vi "Glimpse Image Display Controller.vi"() -> ()   [LabVIEW 2015]
doc: "This widget allows the user to separately adjust the properties of mulltiple, independently displayed image windows. The controller is a stand-alone VI that can run in a separate thread from the program that is producing the images, so that the image display settings can be adjusted whilst other things (e.g., data acquisition) are occurring simultaneously."
uses:
  Image to Display event.ctt
  <vilib>/vision/Image Controls.llb/IMAQ Image.ctl
  GLIMPSE Globals.vi
panel:
  in  "to window":i8=9 min=2 max=9 step=1
  in  "Snapshot":bool
  in  "Presets":T1(array[cluster])=[{"Mem"=FALSE, "Black"=-32500.0, "White"=-25000.0, "Recall"=FALSE}]
  in  "Keep this in corner?":bool=TRUE
  in  "Autosize M":bool
  in  "Autoposition M":bool
  in  "Autoscale M":bool
  in  "Zoom +":bool
  in  "Zoom -":bool
  out "In use":bool
  in  "Auto size":bool
  in  "Auto position":bool
  in  "Autoscale":bool
  out "Window Title":string
  in  "Control image window #":u8(slide)=1 max=1 step=1 scale=0.0..1.0
  out "error out":errorcluster
  out "Black/White Levels temp":cluster{ext, ext}(slide)={1.0, 65535.0} scale=-32767.0..327567.0
  in  "Black/White Levels":cluster{ext, ext}(slide)={1.0, 65535.0} scale=-32767.0..327567.0
  in  "Stop":bool
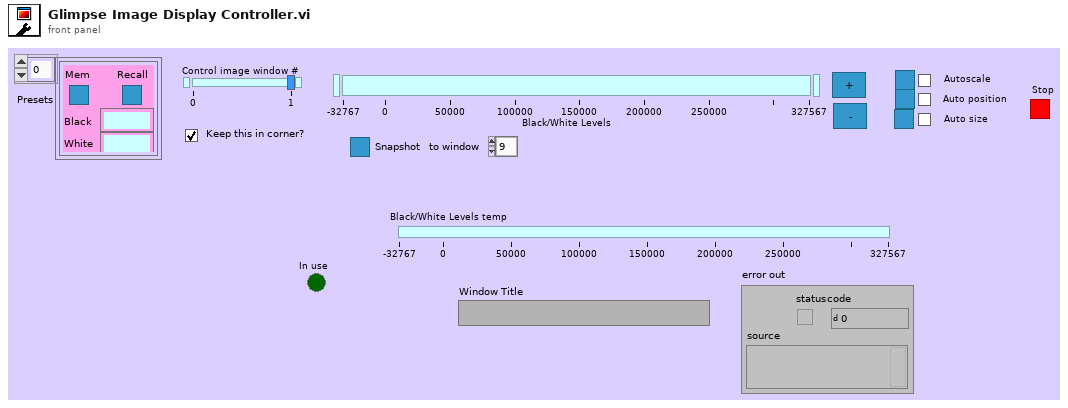
[diagram p1: front panel]
types:
  T1 = cluster{"Mem":bool, "Black":ext, "White":ext, "Recall":bool}[]
  T2 = typedef "Image Type" = u32
  T3 = typedef "IMAQ Image.ctl" = refnum<image>
  T4 = cluster{"Image Type":T2, "Image":T3, "Initialized?":bool, "Window Title":string, "Auto resize?":bool, "Auto position?":bool, "Autoscale?":bool, "Black/White Levels":cluster{ext, ext}, "Scale Min":ext, "Scale Max":ext}
  T5 = typedef "LVRectTypeDef.ctl" = cluster{"Left":i16, "Top":i16, "Right":i16, "Bottom":i16}
  T6 = typedef "Image to Display event.ctt" = cluster{"Image":T3, "Window Title":string, "Window Number":i32, "Image Type":T2, "Quit display controller?":bool}
  T7 = cluster{"Image Type":T2, "Image":T3, "Initialized?":bool, "Window Title":string, "Auto resize?":bool, "Auto position?":bool, "Autoscale?":bool, "Black/White Levels":cluster{ext, ext}, "Scale Min":ext, "Scale Max":ext}[]
  T8 = cluster{"Mem":bool, "Black":ext, "White":ext, "Recall":bool}
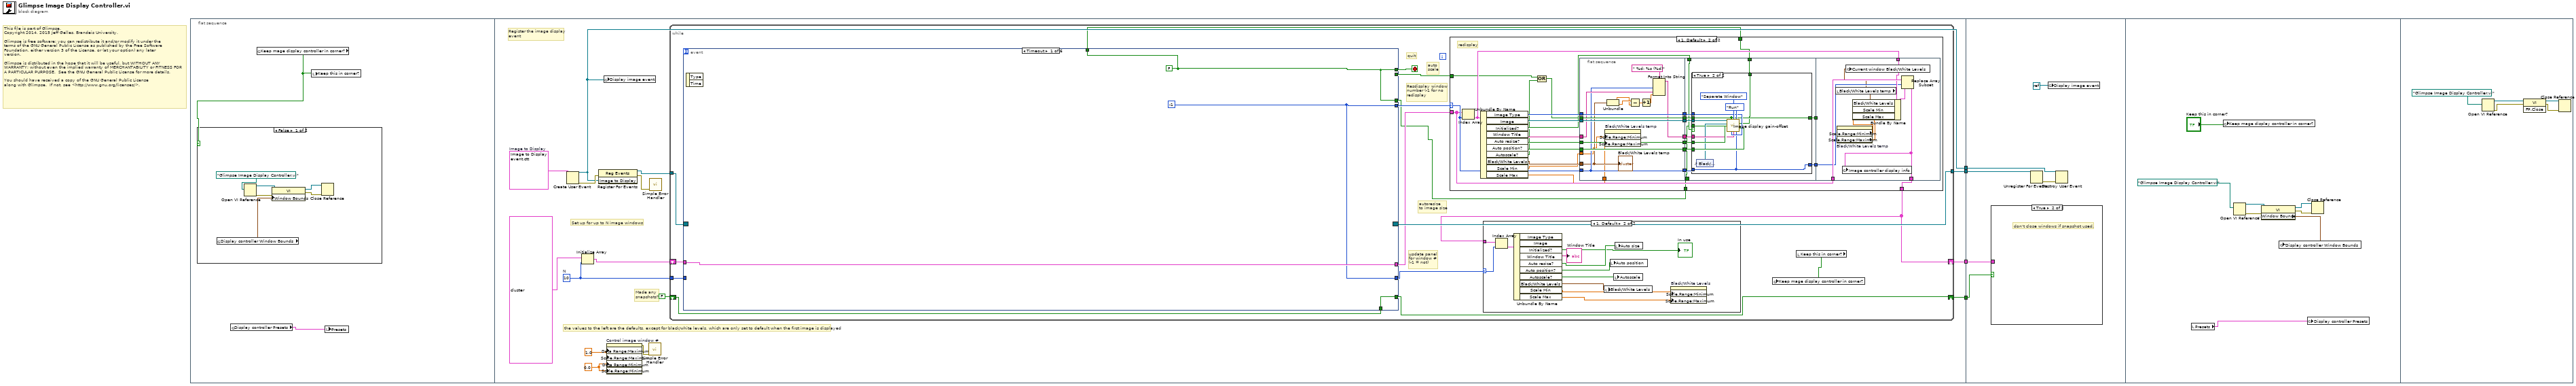
[diagram p0: block diagram]
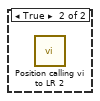
[diagram p2: hidden frame]
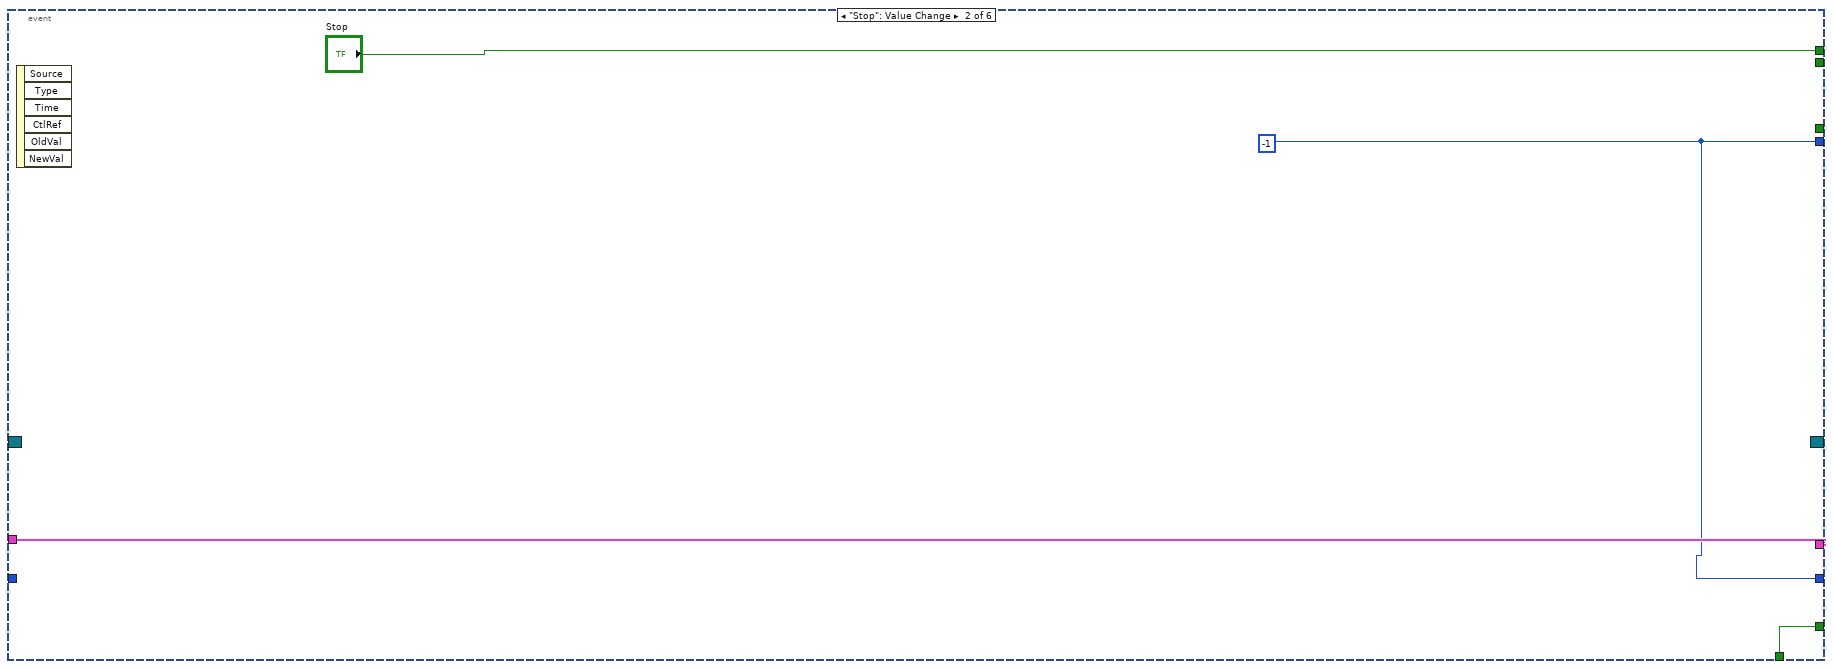
[diagram p6: hidden frame]
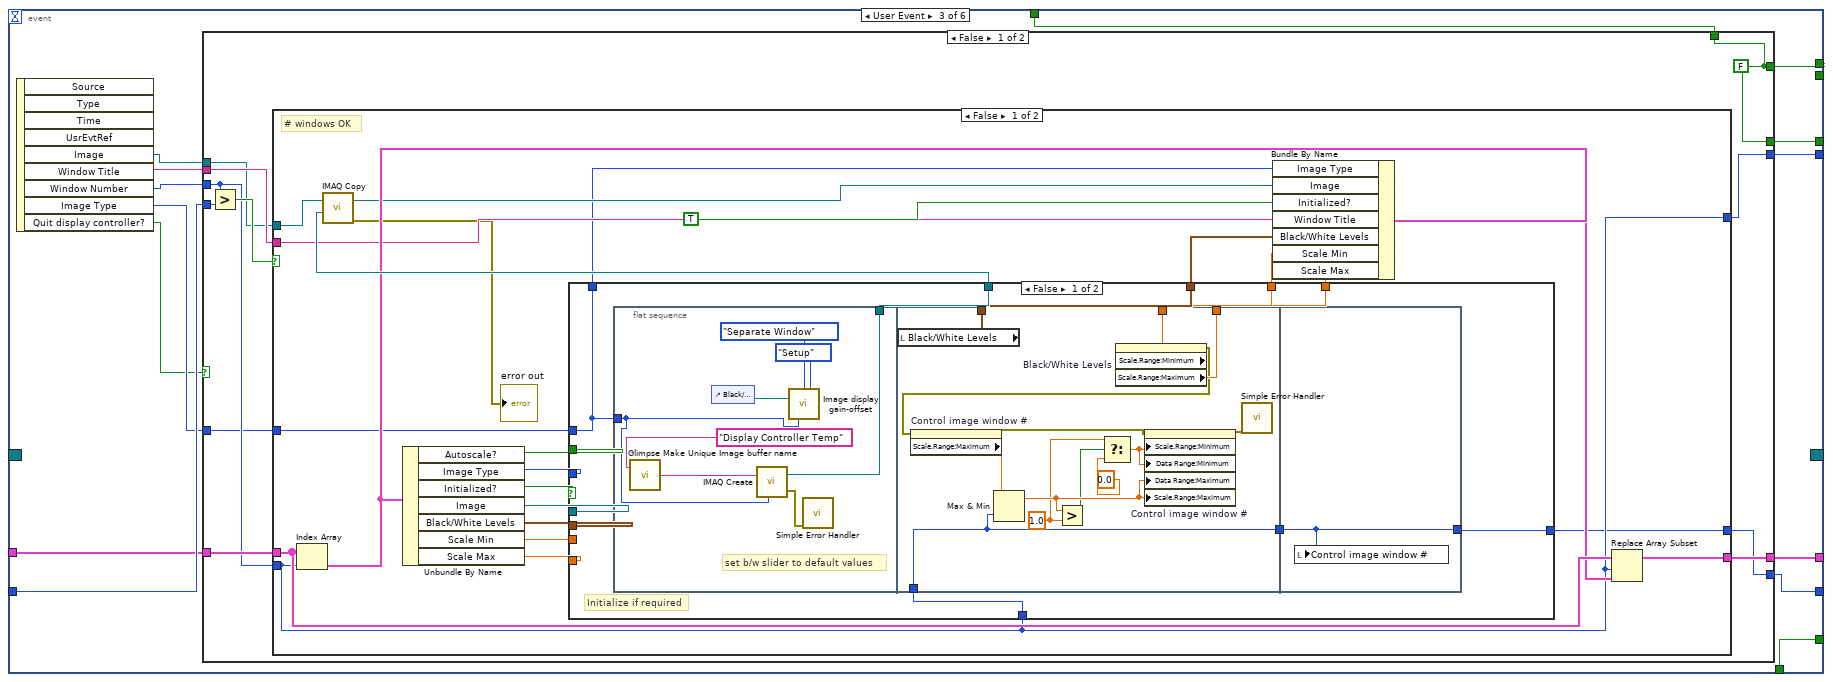
[diagram p7: hidden frame]
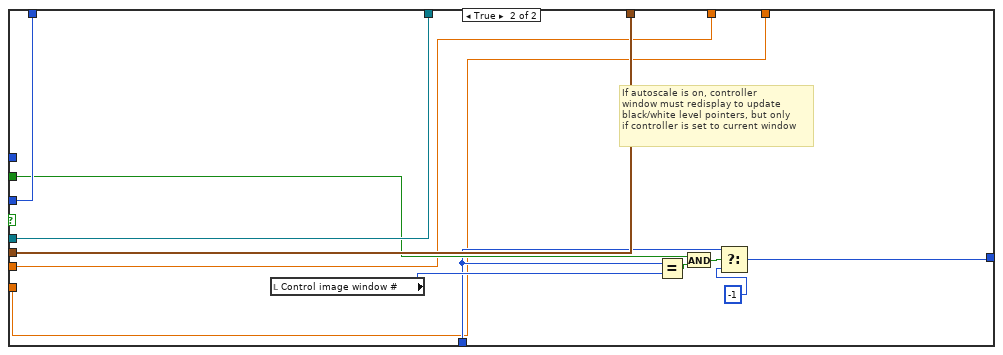
[diagram p8: hidden frame]
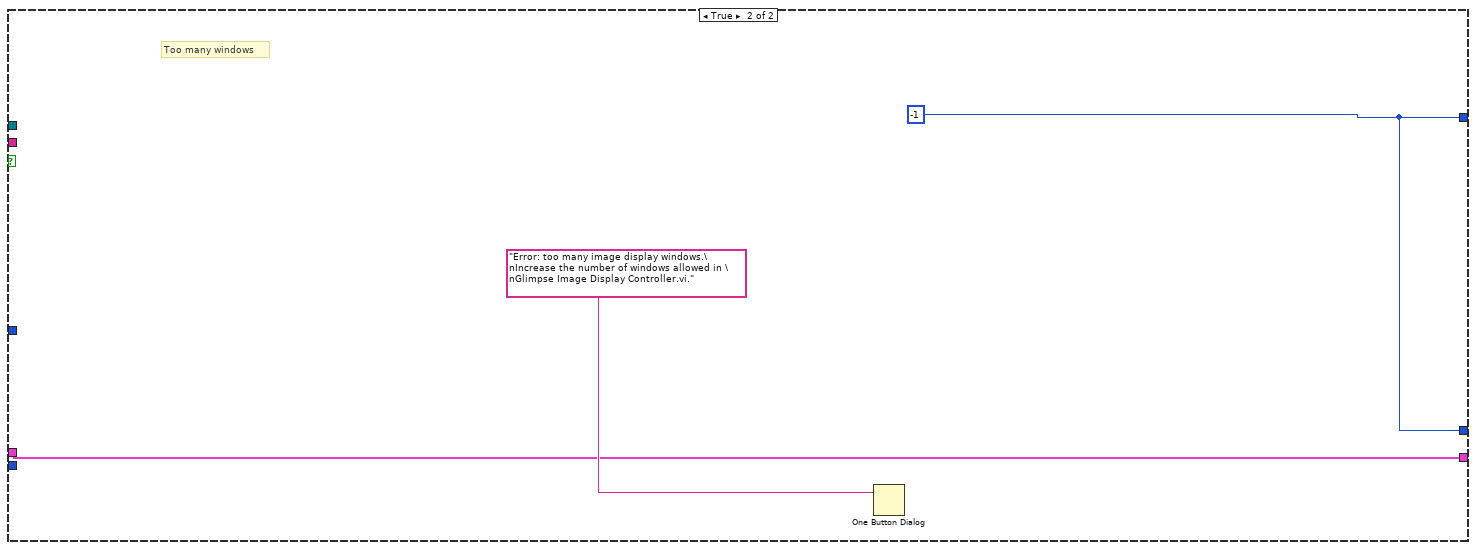
[diagram p9: hidden frame]
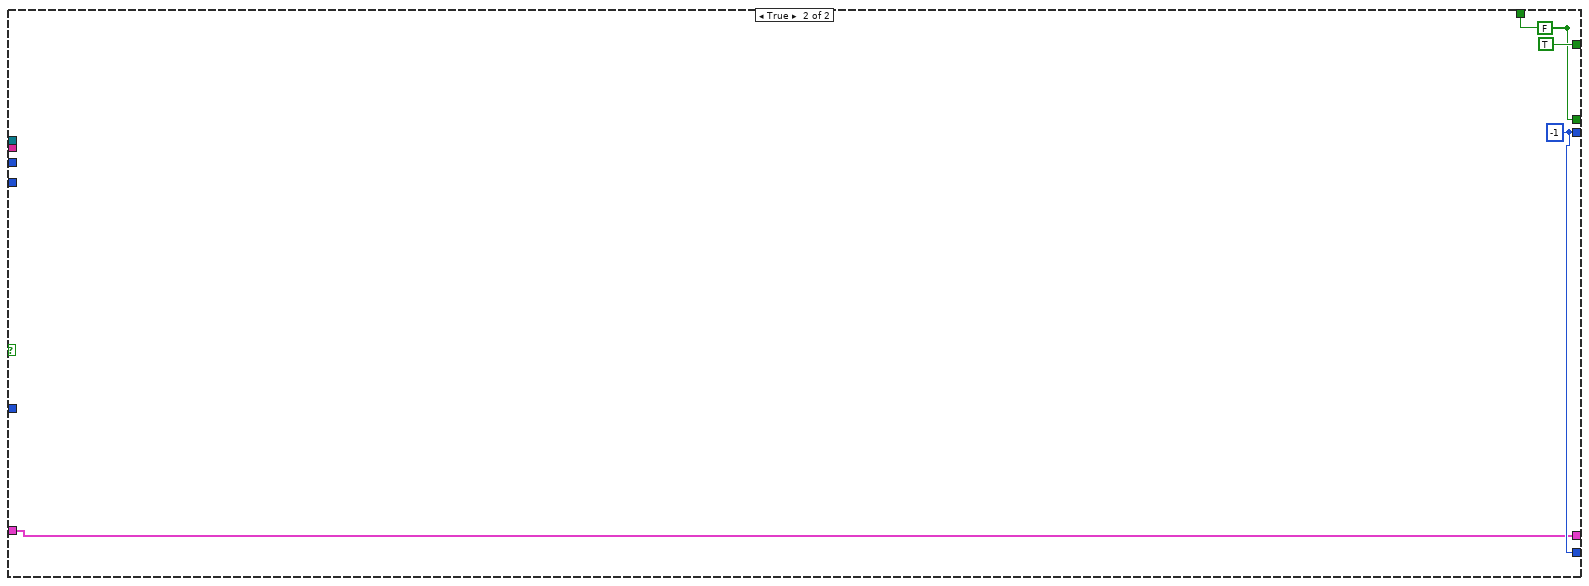
[diagram p10: hidden frame]
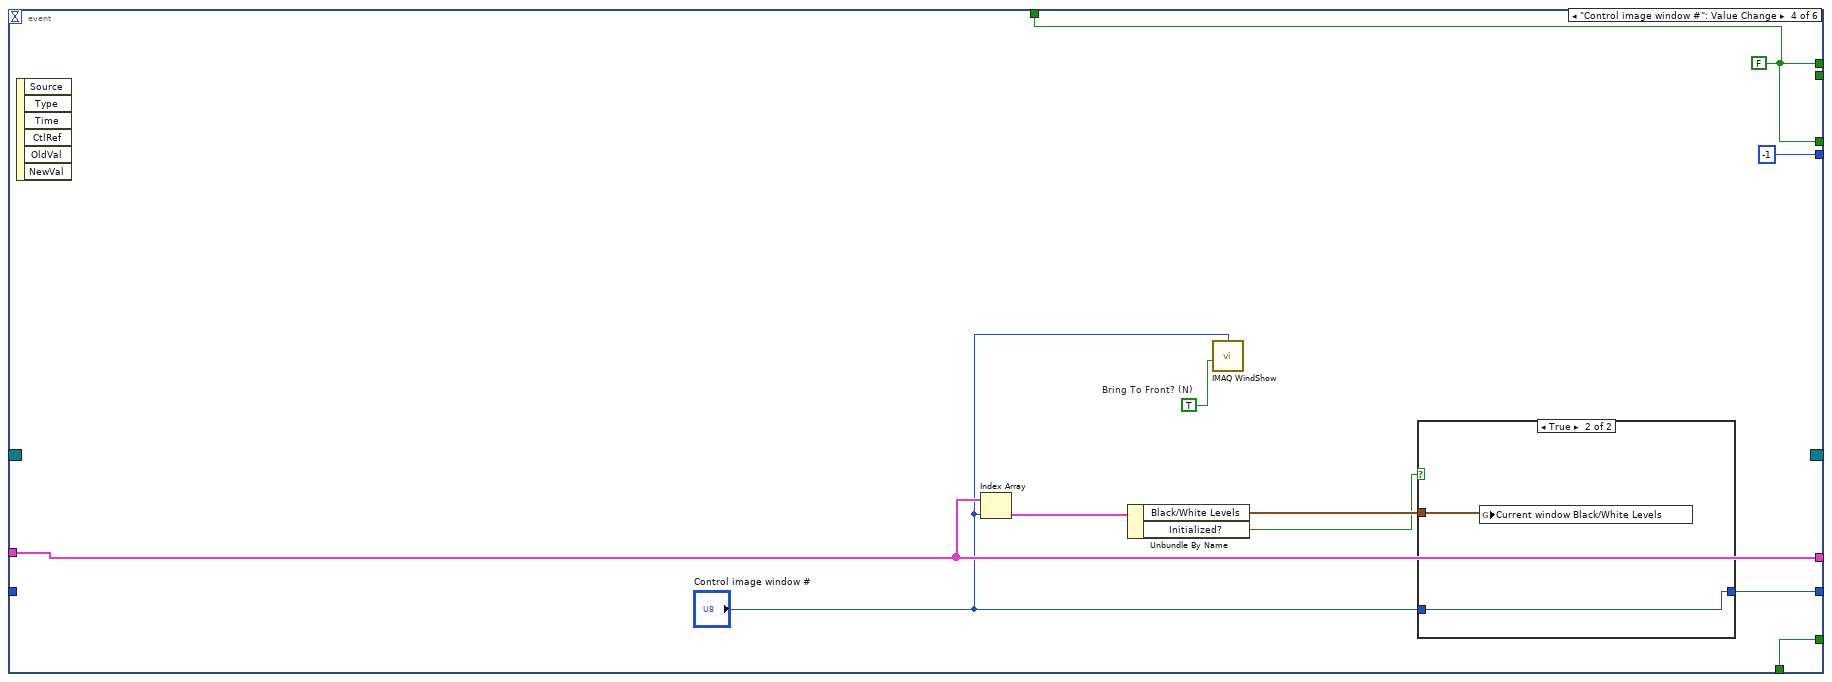
[diagram p11: hidden frame]
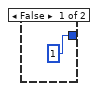
[diagram p12: hidden frame]
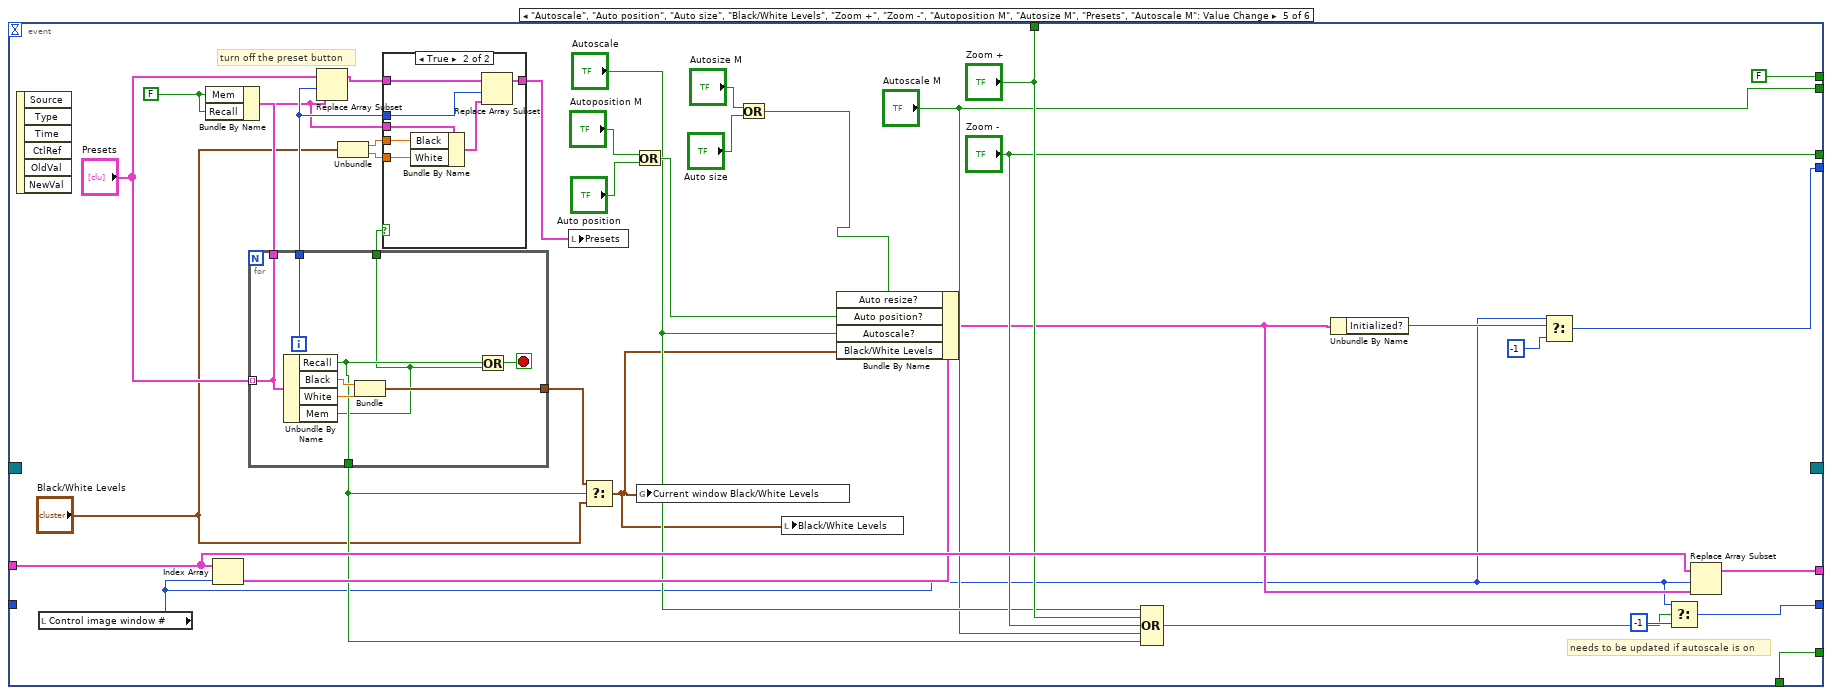
[diagram p13: hidden frame]
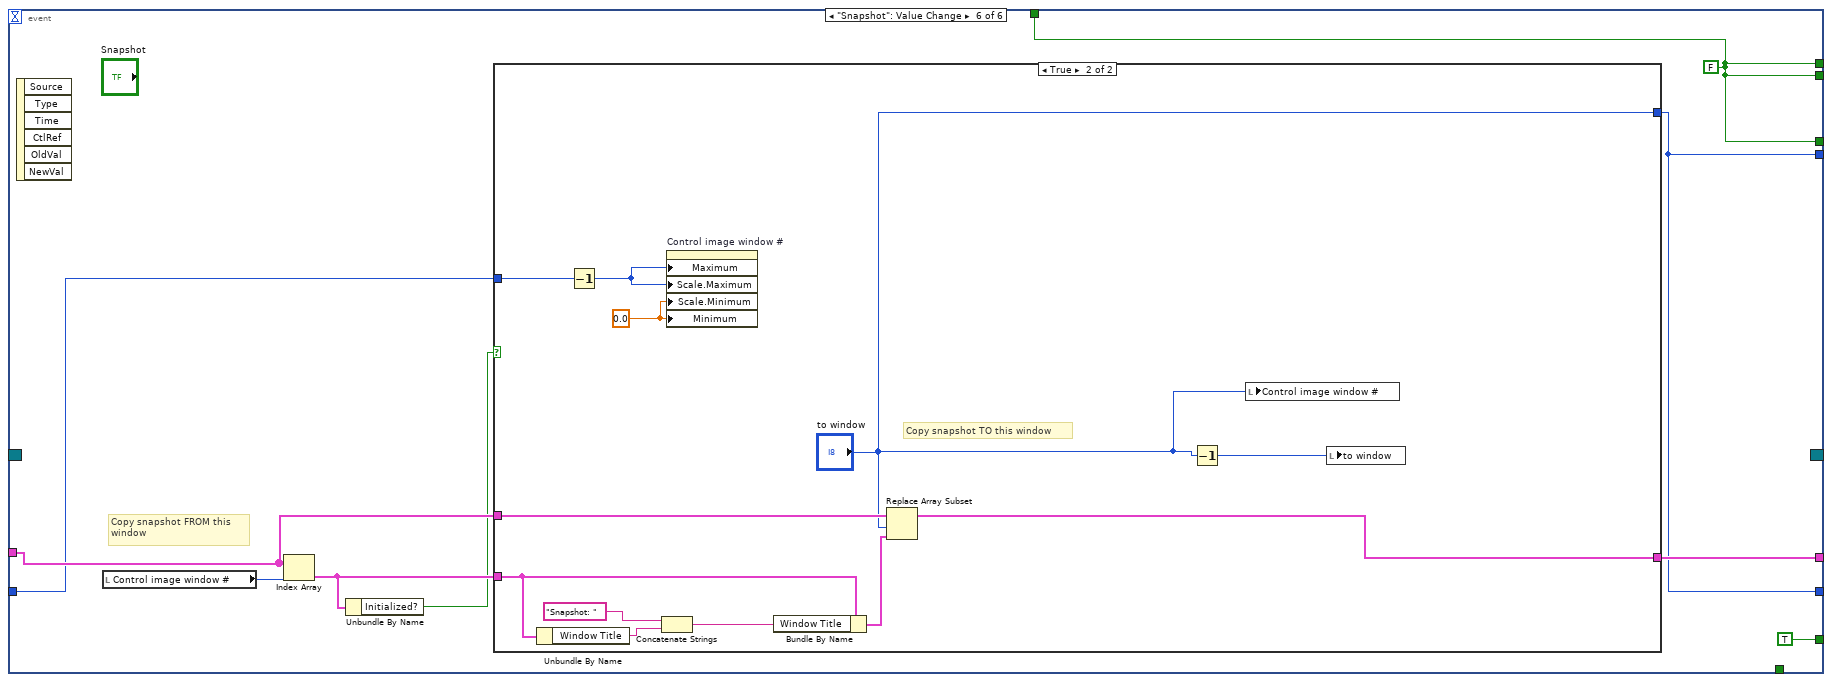
[diagram p15: hidden frame]
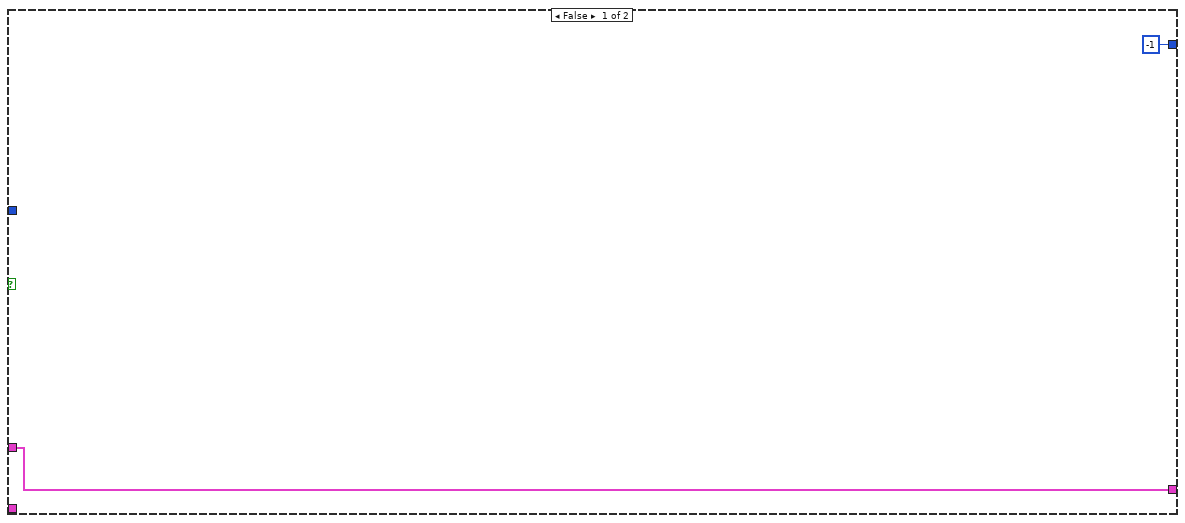
[diagram p16: hidden frame]
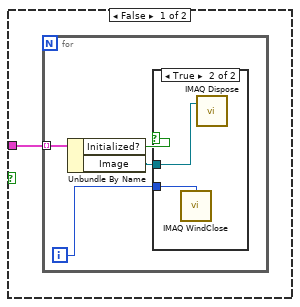
[diagram p17: hidden frame]
diagram:
  # "This file is part of Glimpse. \nCopyright 2014, 2015 Jeff Gelles, Brandeis University.    \n\nGlimpse is free software: you can redistribute it and/or modify it under the \nterms of the GNU General Public License as published by the Free Software \nFoundation, either version 3 of the License, or (at your option) any later \nversion.\n\nGlimpse is distributed in the hope that it will be useful, but WITHOUT ANY \nWARRANTY; without even the implied warranty of MERCHANTABILITY or FITNESS FOR \nA PARTICULAR PURPOSE.  See the GNU General Public License for more details.\n\nYou should have received a copy of the GNU General Public License\nalong with Glimpse.  If not, see <http://www.gnu.org/licenses/>."
  n1 = flat-sequence {
    tunnel: [w24] -> w4
    tunnel: [w18] -> w3
    tunnel: [w19] -> w2
    tunnel: [w13] -> w1
    tunnel: w4 -> [w332]
    tunnel: w3 -> [w330]
    tunnel: w2 -> [w328]
    tunnel: w1 -> [w327]
    frame #0 {
      n2 = global read "GLIMPSE Globals.vi" "Display controller Presets"() -> (w5:T1)
      n3 = global read "GLIMPSE Globals.vi" "Keep mage display controller in corner?"() -> (w6:bool)
      n4 = case shown="False" w6 {
        frame False {
          n5 = global read "GLIMPSE Globals.vi" "Display controller Window Bounds"() -> (w8:T5)
          n6 = Open VI Reference(vi path=path "Glimpse Image Display Controller.vi") -> (vi reference=w12:refnum<vi>, error out=w11:errorcluster)  [unwired: 2 in, 3 out]
          n7 = property class="VI"(reference=w12, error in=w11, "Front Panel Window:Window Bounds"=w8) -> (reference out=w10:refnum<vi>, error out=w9:errorcluster)
          n8 = Close Reference(reference=w10, error in (no error)=w9) -> ()  [unwired: 1 out]
        }
        frame True {
          n9 = call "Position calling vi to LR 2.vi"() -> ()  [unwired: 2 in, 4 out]
        }
      }
      n10 = local write "Keep this in corner?"(w6) -> ()
      n11 = local write "Presets"(w5) -> ()
    }
    frame #1 {
      w16 = 0.0 ("Data Range:Maximum")
      w17 = 1.0 ("Data Range:Maximum")
      w20 = 10  # N
      w23 = T6 {"Image"=refnum, "Window Title"="", "Window Number"=0, "Image Type"=0, "Quit display controller?"=FALSE}  # Image to Display
      # "Made any \nsnapshots?"
      # "the values to the left are the defaults, except for black/white levels, which are only set to default when the first image is displayed"
      # "Set up for up to N image windows"
      # "Register the image display\nevent"
      n12 = Create User Event(user event datatype=w23) -> (user event=w18:refnum<user-event>, error out=w26:errorcluster)  [unwired: 1 in]
      n13 = Initialize Array(T4 {"Image Type"=0, "Image"=refnum, "Initialized?"=FALSE, "Window Title"="", "Auto resize?"=FALSE, "Auto position?"=FALSE, "Autoscale?"=FALSE, "Black/White Levels"={1.0, 2.0}, "Scale Min"=-32767.0, "Scale Max"=327567.0}, w20) -> (w21:T7)
      n14 = register-events(error in=w26, w18) -> (reference out=w27:refnum<event-registration>, error out=w25:errorcluster)  [unwired: 1 in]
      n15 = global write "GLIMPSE Globals.vi" "Display image event"(w18) -> ()
      n16 = property on="Control image window #" class="Slide (strict)"("Data Range:Maximum"=w17, "Scale.Range:Maximum"=w17, "Data Range:Minimum"=w16, "Scale.Range:Minimum"=w16) -> (error out=w15:errorcluster)  [unwired: 2 in, 1 out]
      n17 = call <vilib>:"Simple Error Handler.vi"("error in (no error)"=w15) -> ()  [unwired: 1 in, 8 out]
      n18 = call <vilib>:"Simple Error Handler.vi"("error in (no error)"=w25) -> ()  [unwired: 1 in, 8 out]
      n19 = while {
        shift-right: [w35] -> w19
        shift-left: w21 -> [w40]
        tunnel: w27 -> [w41]
        tunnel: [w37] -> w24
        tunnel: w20 -> [w39]
        shift-right: [w29] -> w13
        shift-left: FALSE ("Stop") -> [w28]
        stop <- w42 stop-if-true
        # "autoresize\nto image size"
        # "auto\nscale"
        # "update panel\nfor window #\n(-1 = not)"
        # "quit"
        # "Resdisplay window\nnumber (-1 for no\nredisplay"
        n20 = event shown="[0] Timeout" {
          selector: w41 -> [_ _ _ _ _ _]
          dyn-events: [_ _ _ _ _ _] -> w37
          timeout: _ -> [_ _ _ _ _ _]
          tunnel: [w134 "Stop" w148 w243 FALSE ("Stop") w310] -> w42
          tunnel: w40 -> [w135 w138 w152 w246 w287 w312]
          tunnel: w39 -> [_ _ w153 _ _ w309]
          tunnel: [w135 w138 w149 w246 w280 w311] -> w36
          tunnel: [w133 w137 w145 -1 ("Window Number") w254 w305] -> w38
          tunnel: [w134 _ w142 w243 "Zoom +" w310] -> w34
          tunnel: [w134 _ w143 w243 "Zoom -" w310] -> w31
          tunnel: [_ _ _ _ "Autoscale M" w310] -> w33
          tunnel: [w133 w137 w141 w239 w257 w305] -> w30
          tunnel: [w132 w136 w140 w238 w251 TRUE ("Stop")] -> w29
          tunnel: w28 -> [w132 w136 w140 w238 w251 _]
          event Timeout {
            w133 = -1 ("Window Number")
            w134 = FALSE ("Stop")
            n21 = event-data() -> ()  [unwired: 3 out]
          }
          event "Stop": Value Change {
            w137 = -1 ("Window Number")
            n22 = event-data() -> ()  [unwired: 7 out]
          }
          event User Event {
            n23 = event-data() -> ("Image"=w146:T3, "Window Title"=w150:string, "Window Number"=w151:i32, "Image Type"=w147:T2, "Quit display controller?"=w144:bool)  [unwired: 5 out]
            n24 = case shown="False" w144 {
              tunnel: w153 -> [w164 _]
              tunnel: w152 -> [w162 w235]
              tunnel: w151 -> [w161 _]
              tunnel: w150 -> [w160 _]
              tunnel: [w159 w235] -> w149
              tunnel: [w154 TRUE] -> w148
              tunnel: w147 -> [w158 _]
              tunnel: w146 -> [w157 _]
              tunnel: [w156 w236] -> w145
              tunnel: [w155 w236] -> w141
              tunnel: [w154 w234] -> w143
              tunnel: [w154 w234] -> w142
              frame False {
                w154 = FALSE
                n25 = Greater?(x=w161, y=w164) -> (0:w163:bool)
                n26 = case shown="False" w163 {
                  tunnel: w162 -> [w179 w232]
                  tunnel: w161 -> [w173 _]
                  tunnel: w157 -> [w185 _]
                  tunnel: w160 -> [w180 _]
                  tunnel: [w165 w232] -> w159
                  tunnel: [w173 w231] -> w156
                  tunnel: w158 -> [w176 _]
                  tunnel: [w172 w231] -> w155
                  frame False {
                    # "# windows OK"
                    n27 = Index Array(array=w179, index=w173) -> (element=w184:T4)
                    n28 = Unbundle By Name(w184) -> ("Autoscale?"=w170:bool, "Image Type"=w181:T2, "Initialized?"=w188:bool, "Image"=w187:T3, "Black/White Levels"=w174:cluster{ext, ext}, "Scale Min"=w167:ext, "Scale Max"=w166:ext)
                    n29 = case shown="False" w188 {
                      tunnel: w181 -> [_ w229]
                      tunnel: [w196 w230] -> w186
                      tunnel: w187 -> [_ w230]
                      tunnel: [w195 w229] -> w177
                      tunnel: w176 -> [w195 _]
                      tunnel: w174 -> [_ w228]
                      tunnel: [w194 w228] -> w171
                      tunnel: w173 -> [w193 w221]
                      tunnel: [w192 w225] -> w172
                      tunnel: w170 -> [_ w226]
                      tunnel: [w191 w220] -> w169
                      tunnel: [w190 w219] -> w168
                      tunnel: w167 -> [_ w220]
                      tunnel: w166 -> [_ w219]
                      frame False {
                        # "Initialize if required"
                        n30 = flat-sequence {
                          tunnel: [w202] -> w196
                          tunnel: w195 -> [w197]
                          tunnel: [w217] -> w194
                          tunnel: w193 -> [w213]
                          tunnel: [w216] -> w191
                          tunnel: [w215] -> w190
                          tunnel: [w213] -> w189
                          tunnel: [w218] -> w192
                          tunnel: w189 -> [w218]
                          frame #0 {
                            # "set b/w slider to default values"
                            n31 = call "Glimpse Make Unique Image buffer name.vi"("Buffer  base name"="Display Controller Temp") -> ("Image Name"=w203:string)  [unwired: 1 out]
                            n32 = control-ref of="Black/White Levels"() -> (w198:refnum<vi>)
                            n33 = call "IMAQ Create"("Image Name"=w203, "Image Type"=w197) -> ("New Image"=w202:T3, "error out"=w201:errorcluster)  [unwired: 2 in, 1 out]
                            n34 = call "Image display gain-offset.vi"("Display Type (s)"=enum16{"Front Panel", "Separate Window"}."Separate Window", "Mode"=enum16{"Setup", "Run"}."Setup", "Black/White Levels Ctl Ref (s)"=w198, "Pixel depth (s)"=w197) -> ()  [unwired: 9 in, 3 out]
                            n35 = call <vilib>:"Simple Error Handler.vi"("error in (no error)"=w201) -> ()  [unwired: 1 in, 8 out]
                          }
                          frame #1 {
                            w206 = 1.0 ("y")
                            n36 = local read "Black/White Levels"() -> (w217:cluster{ext, ext})
                            n37 = property on="Black/White Levels" class="Slide (strict)"() -> (error out=w212:errorcluster, "Scale.Range:Minimum"=w216:dbl, "Scale.Range:Maximum"=w215:dbl)  [unwired: 2 in, 1 out]
                            n38 = property on="Control image window #" class="Slide (strict)"(error in=w212) -> (error out=w211:errorcluster, "Scale.Range:Maximum"=w214:dbl)  [unwired: 1 in, 1 out]
                            n39 = Max & Min(x=w214, y=w213) -> (max(x,y)=w209:dbl)  [unwired: 1 out]
                            n40 = Greater?(x=w209, y=w206) -> (0:w207:bool)
                            n41 = Select(t=w206, s=w207, f=0.0 ("Data Range:Minimum")) -> (s? t:f=w208:dbl)
                            n42 = property on="Control image window #" class="Slide (strict)"(error in=w211, "Scale.Range:Minimum"=w208, "Data Range:Minimum"=w208, "Data Range:Maximum"=w209, "Scale.Range:Maximum"=w209) -> (error out=w210:errorcluster)  [unwired: 1 in, 1 out]
                            n43 = call <vilib>:"Simple Error Handler.vi"("error in (no error)"=w210) -> ()  [unwired: 1 in, 8 out]
                          }
                          frame #2 {
                            n44 = local write "Control image window #"(w218) -> ()
                          }
                        }
                      }
                      frame True {
                        # "If autoscale is on, controller\nwindow must redisplay to update \nblack/white level pointers, but only\nif controller is set to current window"
                        n45 = local read "Control image window #"() -> (w222:u8)
                        n46 = Equal?(x=w221, y=w222) -> (x = y?=w223:bool)
                        n47 = And(x=w226, y=w223) -> (x .and. y?=w224:bool)
                        n48 = Select(t=w221, s=w224, f=-1 ("Window Number")) -> (s? t:f=w225:i32)
                      }
                    }
                    n49 = call "IMAQ Copy"("Image Dst"=w186, "Image Src"=w185) -> ("error out"=→"error out":errorcluster, "Image Dst Out"=w183:T3)  [unwired: 1 in, 3 out]
                    n50 = Bundle By Name(cluster=w184, "Image Type"=w177, "Image"=w183, "Initialized?"=TRUE, "Window Title"=w180, "Black/White Levels"=w171, "Scale Min"=w169, "Scale Max"=w168) -> (w178:T4)
                    n51 = Replace Array Subset(array=w179, new element=w178, index=w173) -> (w165:T7)
                  }
                  frame True {
                    w231 = -1 ("Window Number")
                    # "Too many windows"
                    n52 = One Button Dialog(message="Error: too many image display windows.\nIncrease the number of windows allowed in \nGlimpse Image Display Controller.vi.") -> ()  [unwired: 2 out]
                  }
                }
              }
              frame True {
                w234 = FALSE
                w236 = -1 ("Window Number")
              }
            }
          }
          event "Control image window #": Value Change {
            w242 = TRUE  # Bring To Front? (N)
            w243 = FALSE ("Stop")
            n53 = event-data() -> ()  [unwired: 7 out]
            n54 = Index Array(array=w246, index="Control image window #") -> (element=w245:T4)
            n55 = Unbundle By Name(w245) -> ("Black/White Levels"=w244:cluster{ext, ext}, "Initialized?"=w241:bool)
            n56 = call "IMAQ WindShow"("Bring To Front? (N)"=w242, "Window Number (0...15)"="Control image window #") -> ()  [unwired: 3 in, 4 out]
            n57 = case shown="True" w241 {
              tunnel: w244 -> [_ w250]
              tunnel: "Control image window #" -> [_ w249]
              tunnel: [i8 1 ("Control image window #") w249] -> w239
              frame False {
              }
              frame True {
                n58 = global write "GLIMPSE Globals.vi" "Current window Black/White Levels"(w250) -> ()
              }
            }
          }
          event "Autoscale", "Auto position", "Auto size", "Black/White Levels", "Zoom +", "Zoom -", "Autoposition M", "Autosize M", "Presets", "Autoscale M": Value Change {
            w267 = FALSE ("Select")
            # "turn off the preset button"
            # "needs to be updated if autoscale is on"
            n59 = event-data() -> ()  [unwired: 7 out]
            n60 = local read "Control image window #"() -> (w252:u8)
            n61 = Index Array(array=w287, index=w252) -> (element=w286:T4)
            n62 = for {
              tunnel: "Presets" -> [w299] mode=indexing
              tunnel: [w301] -> w271
              tunnel: [w297] -> w268
              tunnel: [w300] -> w264
              tunnel: [w299] -> w270
              tunnel: [w296] -> w263
              i -> [w300]
              stop <- w298 stop-if-true
              n63 = Unbundle By Name(w299) -> ("Recall"=w297:bool, "Black"=w303:ext, "White"=w302:ext, "Mem"=w296:bool)
              n64 = Bundle("Black"=w303, "White"=w302) -> (w301:cluster{"Black":ext, "White":ext})  [unwired: 1 out]
              n65 = Or(x=w297, y=w296) -> (x .or. y?=w298:bool)
            }
            n66 = Bundle By Name(cluster=w270, "Mem"=w267, "Recall"=w267) -> (w262:T8)
            n67 = Replace Array Subset(array="Presets", new element=w262, index=w264) -> (w266:T1)
            n68 = Unbundle("Black/White Levels") -> (w259:ext, w260:ext)
            n69 = case shown="True" w263 {
              tunnel: w266 -> [w288 w295]
              tunnel: [w288 w294] -> w265
              tunnel: w264 -> [_ w293]
              tunnel: w262 -> [_ w292]
              tunnel: w260 -> [_ w290]
              tunnel: w259 -> [_ w289]
              frame False {
              }
              frame True {
                n70 = Bundle By Name(cluster=w292, "Black"=w289, "White"=w290) -> (w291:T8)
                n71 = Replace Array Subset(array=w295, new element=w291, index=w293) -> (w294:T1)
              }
            }
            n72 = local write "Presets"(w265) -> ()
            n73 = Select(t=w271, s=w268, f="Black/White Levels") -> (s? t:f=w258:cluster{"Black":ext, "White":ext})
            n74 = Or(x="Autoposition M", y="Auto position") -> (x .or. y?=w278:bool)
            n75 = global write "GLIMPSE Globals.vi" "Current window Black/White Levels"(w258) -> ()
            n76 = Or(x="Autosize M", y="Auto size") -> (x .or. y?=w276:bool)
            n77 = local write "Black/White Levels"(w258) -> ()
            n78 = Bundle By Name(cluster=w286, "Auto resize?"=w276, "Auto position?"=w278, "Autoscale?"="Autoscale", "Black/White Levels"=w258) -> (w256:T4)
            n79 = Compound Arithmetic op=OR("Autoscale", "Zoom +", "Zoom -", "Autoscale M", w268) -> (w283:bool)
            n80 = Unbundle By Name(w256) -> ("Initialized?"=w255:bool)
            n81 = Select(t=w252, s=w255, f=-1 ("s? t:f")) -> (s? t:f=w254:i32)
            n82 = Select(t=w252, s=w283, f=-1) -> (s? t:f=w257:i32)
            n83 = Replace Array Subset(array=w287, new element=w256, index=w252) -> (w280:T7)
          }
          event "Snapshot": Value Change {
            w310 = FALSE ("Stop")
            # "Copy snapshot FROM this\nwindow"
            n84 = event-data() -> ()  [unwired: 7 out]
            n85 = local read "Control image window #"() -> (w308:u8)
            n86 = Index Array(array=w312, index=w308) -> (element=w307:T4)
            n87 = Unbundle By Name(w307) -> ("Initialized?"=w306:bool)
            n88 = case shown="True" w306 {
              tunnel: w312 -> [w314 w326]
              tunnel: [w314 w325] -> w311
              tunnel: [i8 -1 ("to window") "to window"] -> w305
              tunnel: w309 -> [_ w319]
              tunnel: w307 -> [_ w316]
              frame False {
              }
              frame True {
                w318 = 0.0 ("Data Entry Limits:Minimum")
                # "Copy snapshot TO this window"
                n89 = Unbundle By Name(w316) -> ("Window Title"=w322:string)
                n90 = Decrement(x=w319) -> (x-1=w317:i32)
                n91 = Concatenate Strings("Snapshot: " ("string"), w322) -> (w321:string)
                n92 = property on="Control image window #" class="Slide (strict)"("Maximum"=w317, "Scale.Maximum"=w317, "Scale.Minimum"=w318, "Minimum"=w318) -> ()  [unwired: 2 in, 2 out]
                n93 = Bundle By Name(cluster=w316, "Window Title"=w321) -> (w320:T4)
                n94 = Replace Array Subset(array=w326, new element=w320, index="to window") -> (w325:T7)
                n95 = Decrement(x="to window") -> (x-1=w315:i8)
                n96 = local write "Control image window #"("to window") -> ()
                n97 = local write "to window"(w315) -> ()
              }
            }
          }
        }
        n98 = case shown="1, Default" w38 {
          selector: w38 -> [_ w78]
          tunnel: w36 -> [w54 w66]
          tunnel: [w54 w63] -> w35
          tunnel: w34 -> [_ w59]
          tunnel: w33 -> [_ w56]
          tunnel: w31 -> [_ w55]
          frame -1 {
          }
          frame 1, Default {
            # "redisplay"
            n99 = Index Array(array=w66, index=w78) -> (element=w64:T4)
            n100 = Unbundle By Name(w64) -> ("Image Type"=w79:T2, "Image"=w81:T3, "Initialized?"=w67:bool, "Window Title"=w77:string, "Auto resize?"=w80:bool, "Auto position?"=w76:bool, "Autoscale?"=w57:bool, "Black/White Levels"=w68:cluster{ext, ext}, "Scale Min"=w61:ext, "Scale Max"=w60:ext)
            n101 = Or(x=w56, y=w57) -> (x .or. y?=w58:bool)
            n102 = flat-sequence {
              tunnel: w76 -> [w93]
              tunnel: w77 -> [w91]
              tunnel: w78 -> [w89]
              tunnel: w79 -> [w94]
              tunnel: w80 -> [w95]
              tunnel: w81 -> [w96]
              tunnel: w58 -> [w97]
              tunnel: [w97] -> w75
              tunnel: [w96] -> w74
              tunnel: [w95] -> w73
              tunnel: [w94] -> w72
              tunnel: [w89] -> w71
              tunnel: [w90] -> w70
              tunnel: [w93] -> w69
              tunnel: w68 -> [w88]
              tunnel: w61 -> [w83]
              tunnel: w60 -> [w82]
              tunnel: w75 -> [w109]
              tunnel: w74 -> [w108]
              tunnel: w73 -> [w107]
              tunnel: w72 -> [w106]
              tunnel: w71 -> [w105]
              tunnel: w70 -> [w104]
              tunnel: w69 -> [w103]
              tunnel: w67 -> [w102]
              tunnel: [w101] -> w65
              tunnel: [w100] -> w62
              tunnel: w59 -> [w99]
              tunnel: w55 -> [w98]
              tunnel: w66 -> [w131]
              tunnel: w65 -> [w129]
              tunnel: w64 -> [w130]
              tunnel: [w125] -> w63
              tunnel: w62 -> [_]
              frame #0 {
                n103 = property on="Black/White Levels temp" class="Slide (strict)"("Scale.Range:Minimum"=w83, "Scale.Range:Maximum"=w82) -> ()  [unwired: 2 in, 2 out]
                n104 = Unbundle(w88) -> (w86:ext, w87:ext)
                n105 = Subtract(x=w87, y=w86) -> (x-y=w85:ext)
                n106 = Increment(x=w85) -> (x+1=w84:ext)
                n107 = Format Into String(format string=" %d: %s (%d)", w89, w91, w84) -> (resulting string=w90:string)  [unwired: 2 in, 1 out]
                "Black/White Levels temp" <- w88
              }
              frame #1 {
                n108 = case shown="True" w102 {
                  tunnel: w109 -> [w110 w115]
                  tunnel: w108 -> [_ w121]
                  tunnel: w107 -> [_ w120]
                  tunnel: w106 -> [_ w119]
                  tunnel: w105 -> [w111 w112]
                  tunnel: w104 -> [_ w118]
                  tunnel: w103 -> [_ w117]
                  tunnel: [w111 w112] -> w101
                  tunnel: [w110 w115] -> w100
                  tunnel: w99 -> [_ w114]
                  tunnel: w98 -> [_ w113]
                  frame False {
                  }
                  frame True {
                    n109 = control-ref of="Black/White Levels temp"() -> (w116:refnum<vi>)
                    n110 = call "Image display gain-offset.vi"("Image In"=w121, "Autoscale?"=w115, "Display Type (s)"=enum16{"Front Panel", "Separate Window"}."Separate Window", "Mode"=enum16{"Setup", "Run"}."Run", "Black/White Levels Ctl Ref (s)"=w116, "Zoom +"=w114, "Auto Resize to Image Size?\n(Window only)"=w120, "Zoom -"=w113, "Auto position\n(Window only)"=w117, "Pixel depth (s)"=w119, "Window Title\n(Window only)"=w118, "Window Number\n(Window only)"=w112) -> ()  [unwired: 1 in, 3 out]
                  }
                }
              }
              frame #2 {
                n111 = local read "Black/White Levels temp"() -> (w124:cluster{ext, ext})
                n112 = property on="Black/White Levels temp" class="Slide (strict)"() -> ("Scale.Range:Minimum"=w127:dbl, "Scale.Range:Maximum"=w126:dbl)  [unwired: 2 in, 2 out]
                n113 = global write "GLIMPSE Globals.vi" "Current window Black/White Levels"(w124) -> ()
                n114 = Bundle By Name(cluster=w130, "Black/White Levels"=w124, "Scale Min"=w127, "Scale Max"=w126) -> (w128:T4)
                n115 = Replace Array Subset(array=w131, new element=w128, index=w129) -> (w125:T7)
                n116 = global write "GLIMPSE Globals.vi" "Image controller display info"(w125) -> ()
              }
            }
          }
        }
        n117 = case shown="1, Default" w30 {
          selector: w30 -> [_ w46]
          tunnel: w35 -> [_ w52]
          frame -1 {
          }
          frame 1, Default {
            n118 = Index Array(array=w52, index=w46) -> (element=w53:T4)
            n119 = Unbundle By Name(w53) -> ("Initialized?"=→"In use":bool, "Window Title"=→"Window Title":string, "Auto resize?"=w49:bool, "Auto position?"=w48:bool, "Autoscale?"=w47:bool, "Black/White Levels"=w50:cluster{ext, ext}, "Scale Min"=w43:ext, "Scale Max"=w44:ext)  [unwired: 2 out]
            n120 = local write "Black/White Levels"(w50) -> ()
            n121 = local write "Auto position"(w48) -> ()
            n122 = local write "Autoscale"(w47) -> ()
            n123 = local write "Auto size"(w49) -> ()
            n124 = property on="Black/White Levels" class="Slide (strict)"("Scale.Range:Minimum"=w43, "Scale.Range:Maximum"=w44) -> ()  [unwired: 2 in, 2 out]
          }
        }
        n125 = local read "Keep this in corner?"() -> (w32:bool)
        n126 = global write "GLIMPSE Globals.vi" "Keep mage display controller in corner?"(w32) -> ()
      }
    }
    frame #2 {
      n127 = case shown="True" w327 {
        tunnel: w328 -> [w333 _]
        frame False {
          n128 = for {
            tunnel: w333 -> [w337] mode=indexing
            i -> [w334]
            n129 = Unbundle By Name(w337) -> ("Initialized?"=w336:bool, "Image"=w335:T3)
            n130 = case shown="True" w336 {
              tunnel: w335 -> [_ w339]
              tunnel: w334 -> [_ w338]
              frame False {
              }
              frame True {
                n131 = call "IMAQ WindClose"("Window Number (0...15)"=w338) -> ()  [unwired: 2 in, 4 out]
                n132 = call "IMAQ Dispose"("Image"=w339) -> ()  [unwired: 2 in, 4 out]
              }
            }
          }
        }
        frame True {
          # "don't close windows if snapshot used."
        }
      }
      n133 = Unregister For Events(event registration refnum=w332) -> (error out=w331:errorcluster)  [unwired: 1 in]
      n134 = global write "GLIMPSE Globals.vi" "Display image event"(refnum<k0> refnum) -> ()
      n135 = Destroy User Event(user event=w330, error in=w331) -> ()  [unwired: 1 out]
    }
    frame #3 {
      n136 = local read "Presets"() -> (w340:T1)
      n137 = global write "GLIMPSE Globals.vi" "Keep mage display controller in corner?"("Keep this in corner?") -> ()
      n138 = Open VI Reference(vi path=path "Glimpse Image Display Controller.vi") -> (vi reference=w346:refnum<vi>, error out=w345:errorcluster)  [unwired: 1 in, 4 out]
      n139 = property class="VI"(reference=w346, error in=w345) -> (reference out=w344:refnum<vi>, error out=w343:errorcluster, "Front Panel Window:Window Bounds"=w342:T5)
      n140 = global write "GLIMPSE Globals.vi" "Display controller Window Bounds"(w342) -> ()
      n141 = global write "GLIMPSE Globals.vi" "Display controller Presets"(w340) -> ()
      n142 = Close Reference(reference=w344, error in (no error)=w343) -> ()  [unwired: 1 out]
    }
    frame #4 {
      n143 = Open VI Reference(vi path=path "Glimpse Image Display Controller.vi") -> (vi reference=w349:refnum<vi>, error out=w350:errorcluster)  [unwired: 1 in, 4 out]
      n144 = invoke class="VI" method="FP.Close"(reference=w349, error in=w350) -> (reference out=w351:refnum<vi>, error out=w352:errorcluster)  [unwired: 1 in, 1 out]
      n145 = Close Reference(reference=w351, error in (no error)=w352) -> ()  [unwired: 1 out]
    }
  }
